vi "FGV_Timer.vi"(8 "error in (no error)":errorcluster, 10 "TargetTime(0)":dbl, 11 "Mode (Start)":enum16{"Start", "GetTime", "Pause", "UnPause"}(ring)) -> (0 "error out":errorcluster, 1 "Paused?":bool, 2 "Elapsed?":bool, 3 "ElapsedTime":dbl)   [LabVIEW 2017]
doc: "Pausable timer based on functional global variable (FGV)"
panel:
  # "INPUTS"
  # "OUTPUTS"
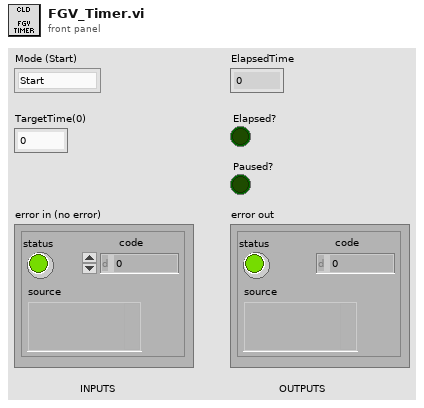
[diagram p1: front panel]
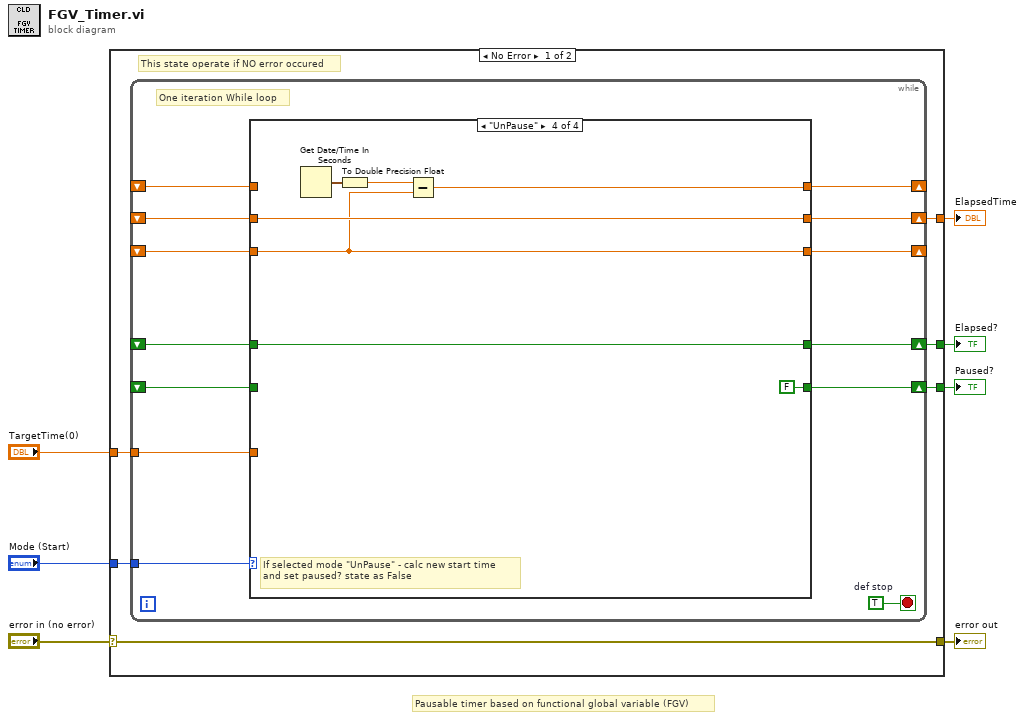
[diagram p0: block diagram]
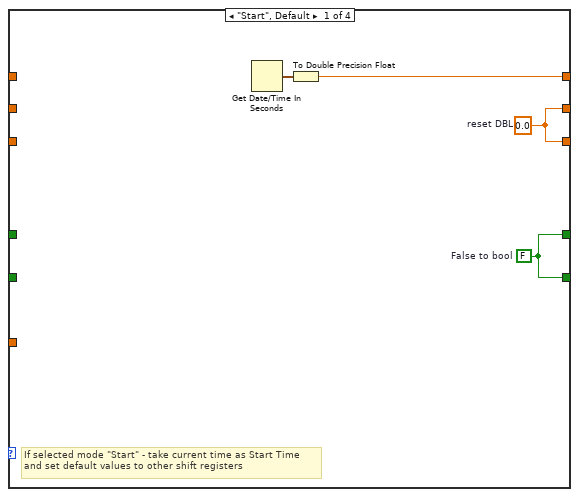
[diagram p2: hidden frame]
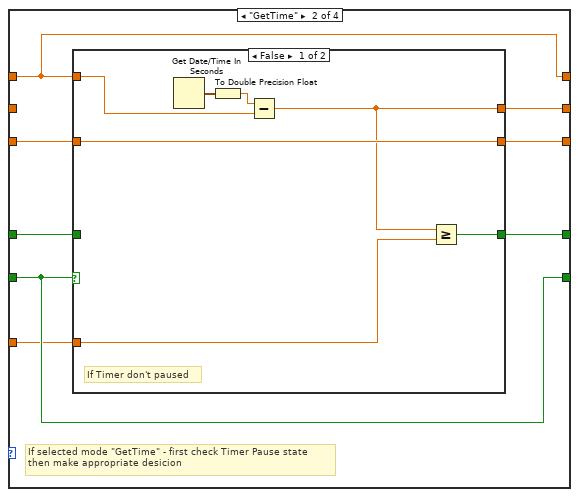
[diagram p3: hidden frame]
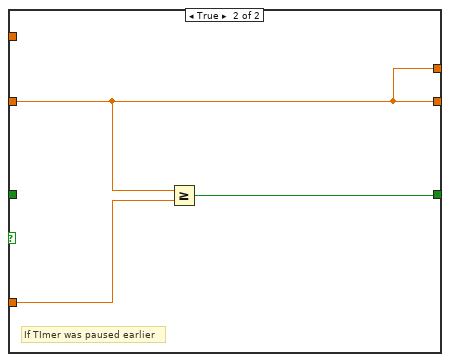
[diagram p4: hidden frame]
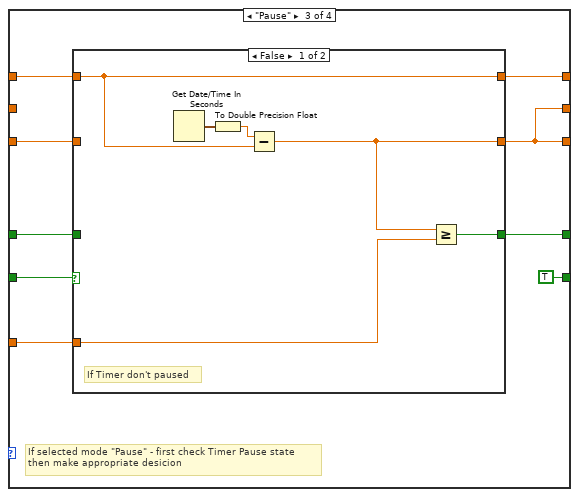
[diagram p5: hidden frame]
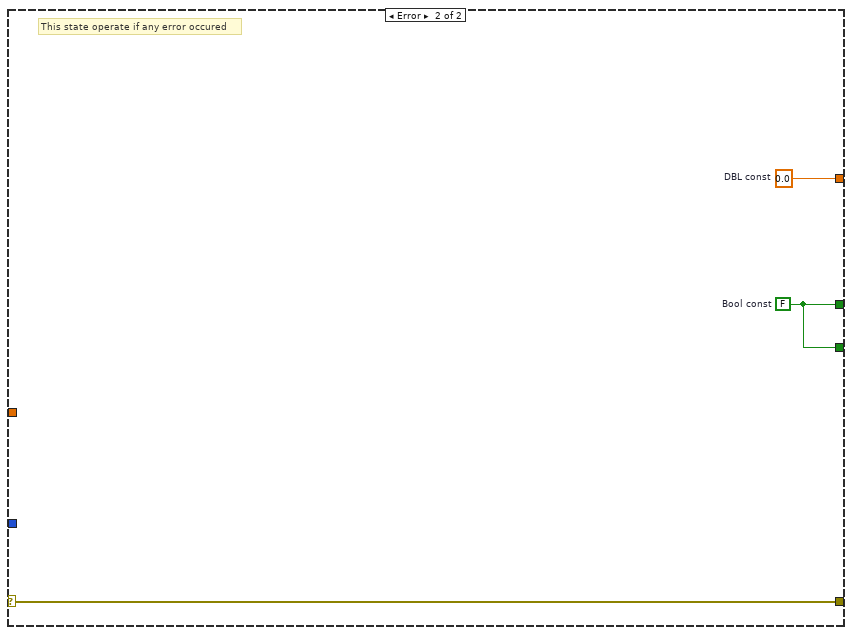
[diagram p7: hidden frame]
diagram:
  # "Pausable timer based on functional global variable (FGV)"
  n1 = case shown="No Error" "error in (no error)" {
    selector: "error in (no error)" -> [w11 w76]
    tunnel: [w11 w76] -> w6
    tunnel: "Mode (Start)" -> [w13 _]
    tunnel: "TargetTime(0)" -> [w12 _]
    tunnel: [w10 w74] -> w3
    tunnel: [w9 w74] -> w2
    tunnel: [w8 w75] -> w1
    frame No Error {
      # "This state operate if NO error occured"
      n2 = while {
        tunnel: w13 -> [w25]
        tunnel: w12 -> [w24]
        shift-right: [w23] -> _
        shift-left: _ -> [w18]
        shift-right: [w22] -> w8
        shift-left: _ -> [w17]
        shift-right: [w21] -> _
        shift-left: _ -> [w16]
        shift-right: [w20] -> w9
        shift-left: _ -> [w15]
        shift-right: [w19] -> w10
        shift-left: _ -> [w14]
        stop <- w26 stop-if-true
        w26 = TRUE  # def stop
        # "One iteration While loop"
        n3 = case shown="\"UnPause\"" w25 {
          tunnel: w24 -> [_ w31 w52 _]
          tunnel: [w29 w33 w49 w71] -> w23
          tunnel: [w28 w32 w50 w70] -> w22
          tunnel: [w28 w37 w50 w69] -> w21
          tunnel: [w27 w35 w55 w68] -> w20
          tunnel: [w27 w34 TRUE ("False to bool") FALSE ("False to bool")] -> w19
          tunnel: w18 -> [_ w33 w53 _]
          tunnel: w17 -> [_ _ _ w70]
          tunnel: w16 -> [_ w38 w57 w69]
          tunnel: w15 -> [_ w36 w56 w68]
          tunnel: w14 -> [_ w34 w54 _]
          frame "Start", Default {
            w27 = FALSE  # False to bool
            w28 = 0.0  # reset DBL
            # "If selected mode \"Start\" - take current time as Start Time\nand set default values to other shift registers"
            n4 = Get Date/Time In Seconds() -> (seconds since 1Jan1904=w30:timestamp)
            n5 = To Double Precision Float(number=w30) -> (double precision float=w29:dbl)
          }
          frame "GetTime" {
            # "If selected mode \"GetTime\" - first check Timer Pause state\nthen make appropriate desicion"
            n6 = case shown="False" w34 {
              tunnel: w38 -> [w42 w48]
              tunnel: [w42 w48] -> w37
              tunnel: w33 -> [w43 _]
              tunnel: w36 -> [_ _]
              tunnel: [w39 w46] -> w35
              tunnel: [w41 w48] -> w32
              tunnel: w31 -> [w40 w47]
              frame False {
                # "If Timer don't paused"
                n7 = Get Date/Time In Seconds() -> (seconds since 1Jan1904=w45:timestamp)
                n8 = To Double Precision Float(number=w45) -> (double precision float=w44:dbl)
                n9 = Subtract(x=w44, y=w43) -> (x-y=w41:dbl)
                n10 = Greater Or Equal?(x=w41, y=w40) -> (x >= y?=w39:bool)
              }
              frame True {
                # "If TImer was paused earlier"
                n11 = Greater Or Equal?(x=w48, y=w47) -> (x >= y?=w46:bool)
              }
            }
          }
          frame "Pause" {
            # "If selected mode \"Pause\" - first check Timer Pause state\nthen make appropriate desicion"
            n12 = case shown="False" w54 {
              tunnel: w57 -> [_ w66]
              tunnel: [w58 w66] -> w50
              tunnel: w53 -> [w59 w64]
              tunnel: w56 -> [_ w65]
              tunnel: [w60 w65] -> w55
              tunnel: w52 -> [w61 _]
              tunnel: [w59 w64] -> w49
              frame False {
                # "If Timer don't paused"
                n13 = Get Date/Time In Seconds() -> (seconds since 1Jan1904=w63:timestamp)
                n14 = To Double Precision Float(number=w63) -> (double precision float=w62:dbl)
                n15 = Subtract(x=w62, y=w59) -> (x-y=w58:dbl)
                n16 = Greater Or Equal?(x=w58, y=w61) -> (x >= y?=w60:bool)
              }
              frame True {
                # "If TImer was paused earlier"
              }
            }
          }
          frame "UnPause" {
            # "If selected mode \"UnPause\" - calc new start time\nand set paused? state as False"
            n17 = Get Date/Time In Seconds() -> (seconds since 1Jan1904=w73:timestamp)
            n18 = To Double Precision Float(number=w73) -> (double precision float=w72:dbl)
            n19 = Subtract(x=w72, y=w69) -> (x-y=w71:dbl)
          }
        }
      }
    }
    frame Error {
      w74 = FALSE  # Bool const
      w75 = 0.0  # DBL const
      # "This state operate if any error occured"
    }
  }
  "error out" <- w6
  "ElapsedTime" <- w1
  "Elapsed?" <- w2
  "Paused?" <- w3
